vi "React.vi"(8 "error in":errorcluster, 9 "Data":u8[](array[numeric]) format="%.0x", 10 "COB ID":u32 format="%.0x", 11 "CAN Task in":refnum<class "CANopen Task Actor.lvclass">) -> (0 "error out":errorcluster, 3 "CAN Task out":refnum<class "CANopen Task Actor.lvclass">)   [LabVIEW 2024, in "CANopen Task Actor.lvlib" / "CANopen Task Actor.lvclass"]
uses:
  CANopen Task Actor.lvclass/CANopen Task Actor.ctl
  CANopen Task Actor.lvclass
  CANopen.lvclass
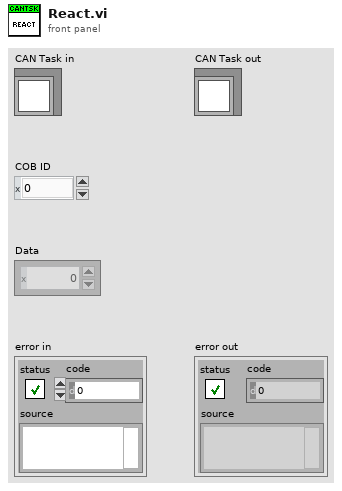
[diagram p1: front panel]
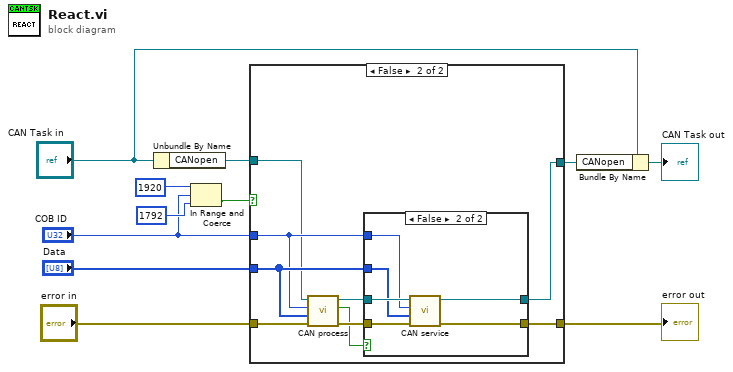
[diagram p0: block diagram]
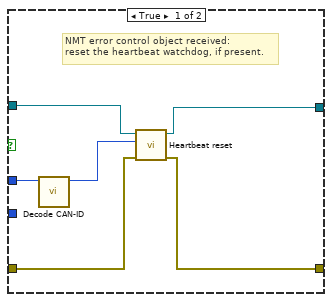
[diagram p2: hidden frame]
diagram:
  n1 = Unbundle By Name("CAN Task in") -> ("CANopen"=w4:refnum<class "CANopen.lvclass">)
  n2 = In Range and Coerce(upper limit=1920 ("x"), x="COB ID", lower limit=1792 ("x")) -> (In Range?=w7:bool)  [unwired: 1 out]
  n3 = case shown="False" w7 {
    tunnel: "error in" -> [w16 w23]
    tunnel: "Data" -> [_ w22]
    tunnel: [w15 w21] -> w5
    tunnel: "COB ID" -> [w17 w20]
    tunnel: w4 -> [w13 w19]
    tunnel: [w12 w18] -> w3
    frame True {
      # "NMT error control object received:\nreset the heartbeat watchdog, if present."
      n4 = call "Decode CAN-ID.vi"("CAN-ID"=w17) -> ("Node ID"=w14:u8)  [unwired: 9 in, 1 out]
      n5 = call "Heartbeat reset.vi"("error in"=w16, "Node ID"=w14, "CANopen in"=w13) -> ("error out"=w15:errorcluster, "CANopen out"=w12:refnum<class "CANopen.lvclass">)  [unwired: 7 in]
    }
    frame False {
      n6 = call "CAN process.vi"("error in (no error)"=w23, "Data"=w22, "COB id"=w20, "CANopen in"=w19) -> ("error out"=w26:errorcluster, "Processed?"=w25:bool, "CANopen out"=w24:refnum<class "CANopen.lvclass">)  [unwired: 5 in]
      n7 = case shown="False" w25 {
        tunnel: w26 -> [w28 w34]
        tunnel: [w28 w33] -> w21
        tunnel: [w27 w32] -> w18
        tunnel: w24 -> [w27 w31]
        tunnel: w20 -> [_ w30]
        tunnel: w22 -> [_ w29]
        frame True {
        }
        frame False {
          n8 = call "CAN service.vi"("error in (no error)"=w34, "Data"=w29, "COB id"=w30, "CANopen in"=w31) -> ("error out"=w33:errorcluster, "CANopen out"=w32:refnum<class "CANopen.lvclass">)  [unwired: 5 in, 1 out]
        }
      }
    }
  }
  "error out" <- w5
  n9 = Bundle By Name(cluster="CAN Task in", "CANopen"=w3) -> (→"CAN Task out":refnum<class "CANopen Task Actor.lvclass">)
